vi "(Incomplete) Elliptic Integral F.vi"(2 "a":dbl=nan format="%.2f", 3 "k":dbl format="%.2f") -> (1 "F(k, a)":dbl format="%.2f")   [LabVIEW 2020, in "NI_Gmath.lvlib"]
doc: "Computes the Legendre elliptic integral of the first kind. It computes the complete elliptic integral of the first kind if you do not wire <B>a</B>."
uses:
  <vilib>/gmath/NI_Gmath.lvlib
  <vilib>/gmath/SpecialFunctions.llb/Incomplete Elliptic Integral F.vi
  <vilib>/gmath/SpecialFunctions.llb/Complete Elliptic Integral K.vi
panel:
  # "This VI is obsolete !!!\nYou should replace this VI in your diagram with the \nElliptic Integral of the 1st kind VI.\n\nNOTE:   Please be aware that the new Elliptic Integral of\n             the 1st kind VI is a polymorphic VI. If you leave \n             the a input of this obsolete VI unwired, please use \n             the Complete Elliptic Integral K instance of the \n             new Elliptic Integral of the 1st kind VI."
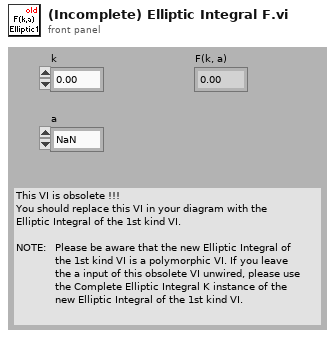
[diagram p1: front panel]
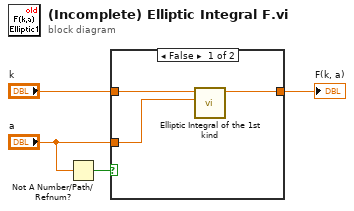
[diagram p0: block diagram]
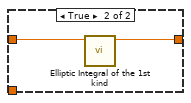
[diagram p2: hidden frame]
diagram:
  n1 = Not A Number/Path/Refnum?(number/path/refnum="a") -> (NaN/Path/Refnum?=w4:bool)
  n2 = case shown="False" w4 {
    tunnel: "a" -> [w6 _]
    tunnel: "k" -> [w7 w9]
    tunnel: [w5 w8] -> w1
    frame False {
      n3 = call-poly <vilib>:"Elliptic Integral of the 1st kind.vi"("a"=w6, "k"=w7) -> ("F(k, a)"=w5:dbl)  [unwired: 9 in]
    }
    frame True {
      n4 = call-poly <vilib>:"Elliptic Integral of the 1st kind.vi"("k"=w9) -> ("K(k)"=w8:dbl)  [unwired: 10 in]
    }
  }
  "F(k, a)" <- w1
